vi "SendLocalMsg.vi"(0 "reference in":refnum<class "MessageInterface.lvclass">, 1 "receiver process":string, 5 "name":string, 7 "value":string, 9 "timeout (25000 ms)":i32=25000, 11 "error in (no error)":errorcluster) -> (4 "reference out":refnum<class "MessageInterface.lvclass">, 10 "timed out?":bool, 15 "error out":errorcluster)   [LabVIEW 2019, in "MessageInterface.lvclass"]
uses:
  MessageInterface.lvclass
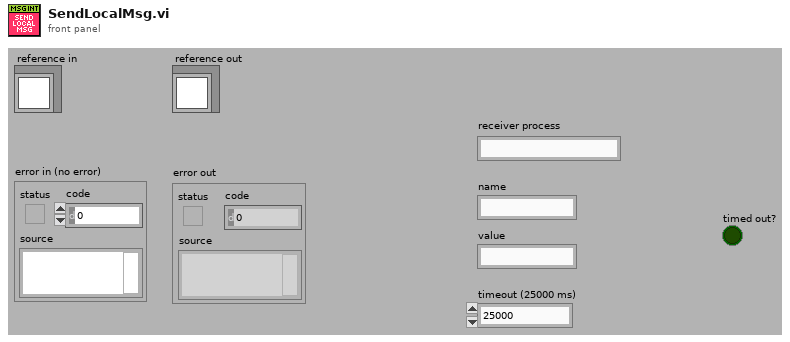
[diagram p1: front panel]
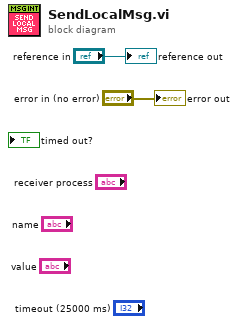
[diagram p0: block diagram]
diagram:
  "error out" <- "error in (no error)"
  "reference out" <- "reference in"
